vi "Update Messages.vi"(8 "error in (no error)":errorcluster, 10 "Message Info":T1, 11 "Data Value Reference in":T2) -> (0 "error out":errorcluster, 2 "PLC MES Error":bool, 3 "Data Value Reference out":T2)   [LabVIEW 2023]
uses:
  <vilib>/Noffz/UTP IO/UTP IO Library/Typedefs/Session Handle.ctl
  <vilib>/Noffz/UTP IO/UTP IO Library/UTP IO Pool Session.lvclass
  MessageInfo.ctl
  <vilib>/Noffz/UTP IO/UTP IO Library/methods/poly/plc/Write PLC Variable (String).vi
  <vilib>/Noffz/UTP IO/UTP IO Library/methods/poly/plc/Write PLC Variable (Boolean).vi
  <vilib>/Noffz/UTP IO/UTP IO Library/methods/poly/plc/Write PLC Variable (I16).vi
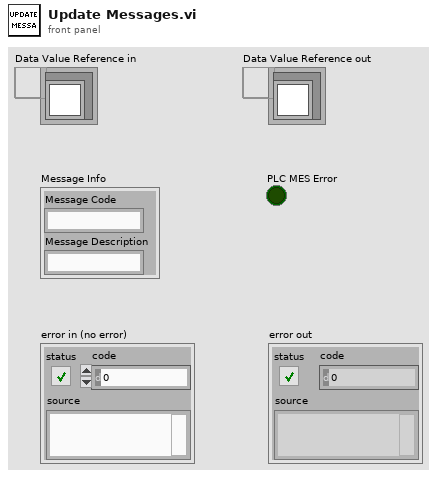
[diagram p1: front panel]
types:
  T1 = typedef "MessageInfo.ctl" = cluster{"Message Code":string, "Message Description":string}
  T2 = typedef "UTP IO Library.lvlib/UTP IO Pool Session.lvclass/Session Handle.ctl" = refnum<data-value>
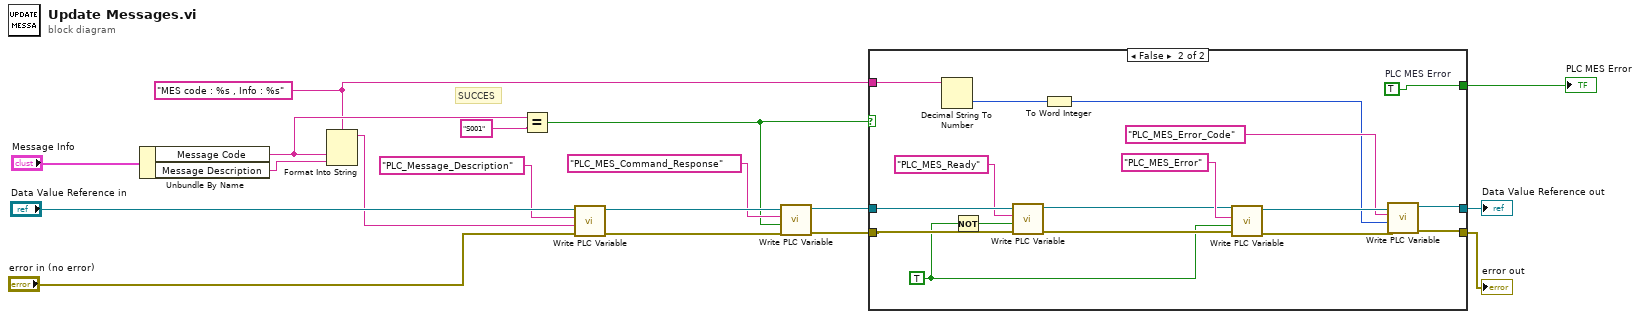
[diagram p0: block diagram]
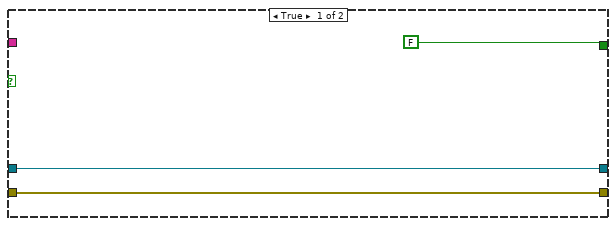
[diagram p2: hidden frame]
diagram:
  w2 = "MES code : %s , Info : %s" ("format string")
  # "SUCCES"
  n1 = Unbundle By Name("Message Info") -> ("Message Code"=w13:string, "Message Description"=w15:string)
  n2 = Format Into String(format string=w2, w13, w15) -> (resulting string=w14:string)  [unwired: 2 in, 1 out]
  n3 = Equal?(x=w13, y="S001") -> (x = y?=w7:bool)
  n4 = call-poly <vilib>:"Write PLC Variable.vi"("error in (no error)"="error in (no error)", "value"=w14, "variable name"="PLC_Message_Description", "UTP IO Session in"="Data Value Reference in") -> ("error out"=w10:errorcluster, "UTP IO Session out"=w12:T2)  [unwired: 6 in]
  n5 = call-poly <vilib>:"Write PLC Variable.vi"("error in (no error)"=w10, "value"=w7, "variable name"="PLC_MES_Command_Response", "UTP IO Session in"=w12) -> ("error out"=w4:errorcluster, "UTP IO Session out"=w6:T2)  [unwired: 6 in]
  n6 = case shown="False" w7 {
    tunnel: w6 -> [w21 w26]
    tunnel: [w21 w37] -> w5
    tunnel: w4 -> [w20 w28]
    tunnel: [w20 w35] -> w3
    tunnel: w2 -> [_ w32]
    tunnel: [FALSE ("PLC MES Error") w29] -> w1
    frame True {
    }
    frame False {
      w29 = TRUE  # PLC MES Error
      w23 = TRUE ("value")
      n7 = Decimal String To Number(string=w32) -> (number=w30:i32)  [unwired: 2 in, 1 out]
      n8 = Not(x=w23) -> (.not. x?=w22:bool)
      n9 = call-poly <vilib>:"Write PLC Variable.vi"("error in (no error)"=w28, "value"=w22, "variable name"="PLC_MES_Ready", "UTP IO Session in"=w26) -> ("error out"=w27:errorcluster, "UTP IO Session out"=w25:T2)  [unwired: 6 in]
      n10 = To Word Integer(number=w30) -> (16bit integer=w31:i16)
      n11 = call-poly <vilib>:"Write PLC Variable.vi"("error in (no error)"=w27, "value"=w23, "variable name"="PLC_MES_Error", "UTP IO Session in"=w25) -> ("error out"=w36:errorcluster, "UTP IO Session out"=w38:T2)  [unwired: 6 in]
      n12 = call-poly <vilib>:"Write PLC Variable.vi"("error in (no error)"=w36, "value"=w31, "variable name"="PLC_MES_Error_Code", "UTP IO Session in"=w38) -> ("error out"=w35:errorcluster, "UTP IO Session out"=w37:T2)  [unwired: 6 in]
    }
  }
  "error out" <- w3
  "Data Value Reference out" <- w5
  "PLC MES Error" <- w1
